vi "Read Data Based on Conrol.vi"(8 "error in (no error)":errorcluster, 10 "Data Refnum":refnum<vi>, 11 "File Refnum":T1) -> (0 "error out":errorcluster, 3 "dup File Refnum":T1)   [LabVIEW 2013]
uses:
  <vilib>/Utility/config.llb/Config Data RefNum.ctl
  <vilib>/Utility/config.llb/NI_LVConfig.lvlib
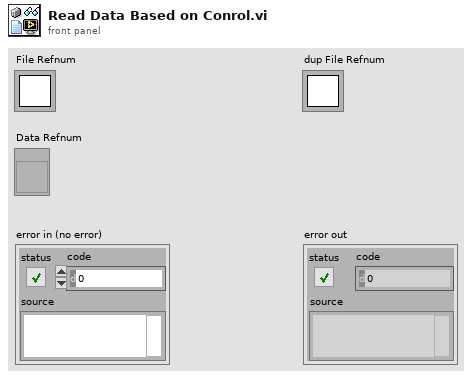
[diagram p1: front panel]
types:
  T1 = typedef "NI_LVConfig.lvlib/Config Data RefNum.ctl" = refnum<k1>
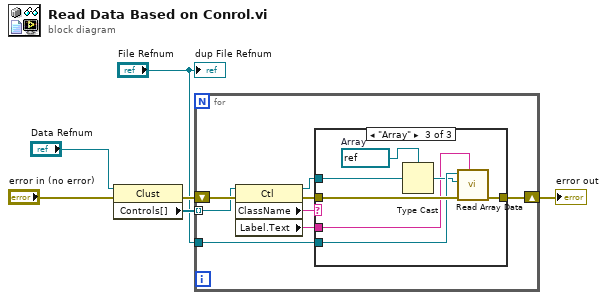
[diagram p0: block diagram]
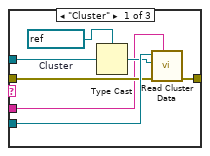
[diagram p2: hidden frame]
diagram:
  n1 = property class="Clust"(reference="Data Refnum", error in="error in (no error)") -> (error out=w4:errorcluster, "Controls[]"=w5:refnum<vi>[])  [unwired: 1 out]
  n2 = for {
    tunnel: w5 -> [w11] mode=indexing
    shift-right: [w14] -> w2
    shift-left: w4 -> [w12]
    tunnel: "File Refnum" -> [w13]
    n3 = property class="Ctl"(reference=w11, error in=w12) -> (reference out=w8:refnum<vi>, error out=w9:errorcluster, "ClassName"=w10:string, "Label.Text"=w7:string)
    n4 = case shown="\"Array\"" w10 {
      tunnel: w9 -> [w17 w22 w29]
      tunnel: w13 -> [w21 _ w27]
      tunnel: [w20 w22 w28] -> w14
      tunnel: w8 -> [w19 _ w26]
      tunnel: w7 -> [w15 _ w23]
      frame "Cluster" {
        w18 = refnum<vi> refnum  # Cluster
        n5 = Type Cast(type=w18, x=w19) -> (*(type *) &x=w16:refnum<vi>)
        n6 = call "Read Cluster Data.vi"("Section Name"=w15, "error in (no error)"=w17, "Clust Refnum"=w16, "File Refnum"=w21) -> ("error out"=w20:errorcluster)  [unwired: 6 in, 1 out]
      }
      frame "others", Default {
      }
      frame "Array" {
        w25 = refnum<vi> refnum  # Array
        n7 = Type Cast(type=w25, x=w26) -> (*(type *) &x=w24:refnum<vi>)
        n8 = call "Read Array Data.vi"("Section Name"=w23, "error in (no error)"=w29, "Arr Refnum"=w24, "File Refnum"=w27) -> ("error out"=w28:errorcluster)  [unwired: 7 in]
      }
    }
  }
  "error out" <- w2
  "dup File Refnum" <- "File Refnum"
